vi "WSVCAP SHL Host LL I2C Build DUT Mask.vi"(0 "DUT":T2, 5 "Device":T1) -> (4 "Socket Mask Set [U64]":u64[](array[numeric]) format="%012x", 8 "DUT Mask":bool[][](array[boolean]))   [LabVIEW 2012]
uses:
  Type Defs/WSVCAP SHL DUT Number Enum.ctl
  Type Defs/WSVCAP SHL I2C Device Enum.ctl
panel:
  # "DUT 01"
  # "DUT 02"
  # "DUT 03"
  # "DUT 04"
  # "DUT 05"
  # "DUT 06"
  # "DUT 07"
  # "DUT 08"
  # "DUT 09"
  # "DUT 10"
  # "DUT 11"
  # "DUT 12"
  # "DUT 13"
  # "DUT 14"
  # "DUT 15"
  # "DUT 16"
  # "DUT 17"
  # "DUT 18"
  # "DUT 19"
  # "DUT 20"
  # "DUT 21"
  # "DUT 22"
  # "DUT 23"
  # "DUT 24"
  # "DUT 25"
  # "DUT 26"
  # "DUT 27"
  # "DUT 28"
  # "DUT 29"
  # "DUT 30"
  # "DUT 31"
  # "DUT 32"
  # "DUT 33"
  # "DUT 34"
  # "DUT 35"
  # "DUT 36"
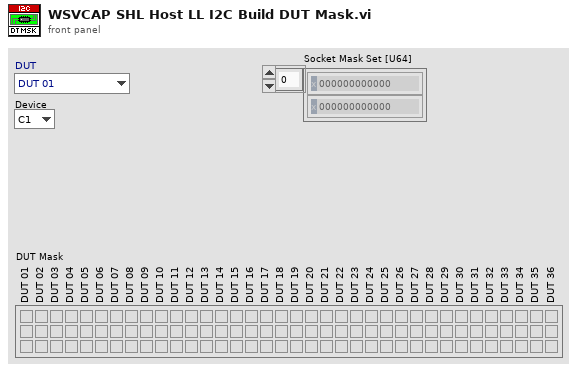
[diagram p1: front panel]
types:
  T1 = typedef "WSVCAP SHL I2C Device Enum.ctl" = enum16{"C1", "C2", "C3"}
  T2 = typedef "WSVCAP SHL DUT Number Enum.ctl" = enum16{"DUT 01", "DUT 02", "DUT 03", "DUT 04", "DUT 05", "DUT 06", "DUT 07", "DUT 08", "DUT 09", "DUT 10", "DUT 11", "DUT 12", "DUT 13", "DUT 14", "DUT 15", "DUT 16", "DUT 17", "DUT 18", "DUT 19", "DUT 20", "DUT 21", "DUT 22", "DUT 23", "DUT 24", "DUT 25", "DUT 26", "DUT 27", "DUT 28", "DUT 29", "DUT 30", "DUT 31", "DUT 32", "DUT 33", "DUT 34", "DUT 35", "DUT 36"}
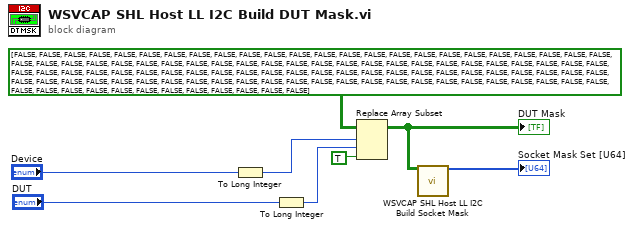
[diagram p0: block diagram]
diagram:
  n1 = To Long Integer(number="Device") -> (32bit integer=w3:i32)
  n2 = To Long Integer(number="DUT") -> (32bit integer=w5:i32)
  n3 = Replace Array Subset(array=bool[][] [[FALSE, FALSE, FALSE, FALSE, FALSE, FALSE, FALSE, FALSE, FALSE, FALSE, FALSE, FALSE, FALSE, FALSE, FALSE, FALSE, FALSE, FALSE, FALSE, FALSE, FALSE, FALSE, FALSE, FALSE, FALSE, FALSE, FALSE, FALSE, FALSE, FALSE, FALSE, FALSE, FALSE, FALSE, FALSE, FALSE], [FALSE, FALSE, FALSE, FALSE, FALSE, FALSE, FALSE, FALSE, FALSE, FALSE, FALSE, FALSE, FALSE, FALSE, FALSE, FALSE, FALSE, FALSE, FALSE, FALSE, FALSE, FALSE, FALSE, FALSE, FALSE, FALSE, FALSE, FALSE, FALSE, FALSE, FALSE, FALSE, FALSE, FALSE, FALSE, FALSE], [FALSE, FALSE, FALSE, FALSE, FALSE, FALSE, FALSE, FALSE, FALSE, FALSE, FALSE, FALSE, FALSE, FALSE, FALSE, FALSE, FALSE, FALSE, FALSE, FALSE, FALSE, FALSE, FALSE, FALSE, FALSE, FALSE, FALSE, FALSE, FALSE, FALSE, FALSE, FALSE, FALSE, FALSE, FALSE, FALSE]], new element=TRUE, index (row)=w3, index (col)=w5) -> (w7:bool[][])
  "DUT Mask" <- w7
  n4 = call "WSVCAP SHL Host LL I2C Build Socket Mask.vi"("DUT Mask Array"=w7) -> ("Socket Mask Set [U64]"=→"Socket Mask Set [U64]":u64[])  [unwired: 14 in]
